vi "FieldMain.vi"() -> ()   [LabVIEW 2014]
uses:
  <vilib>/picture/3D Picture Control/Object/Create Object (drawable).vi
  <vilib>/picture/3D Picture Control/Object/Add Object (no reference).vi
  <vilib>/picture/3D Picture Control/NI_3D Picture Control.lvlib
panel:
  in  "Stopp":bool
  out "3D-Bild":refnum<vi>(3d-picture)
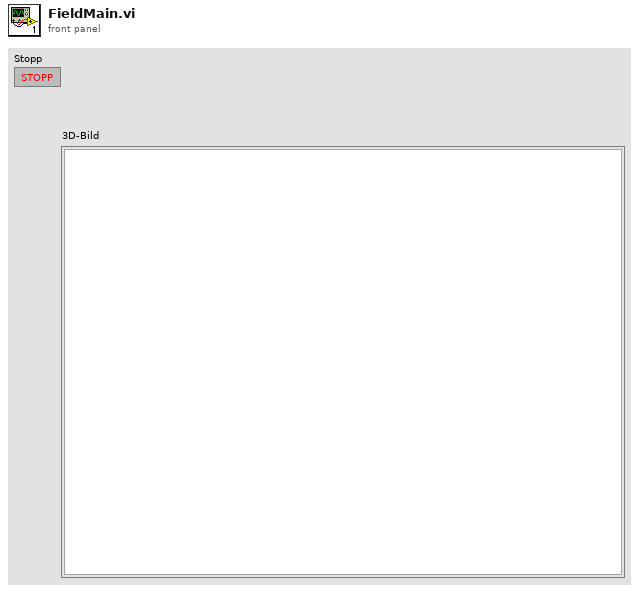
[diagram p1: front panel]
types:
  T1 = cluster{"Red":sgl, "Green":sgl, "Blue":sgl, "Alpha":sgl}
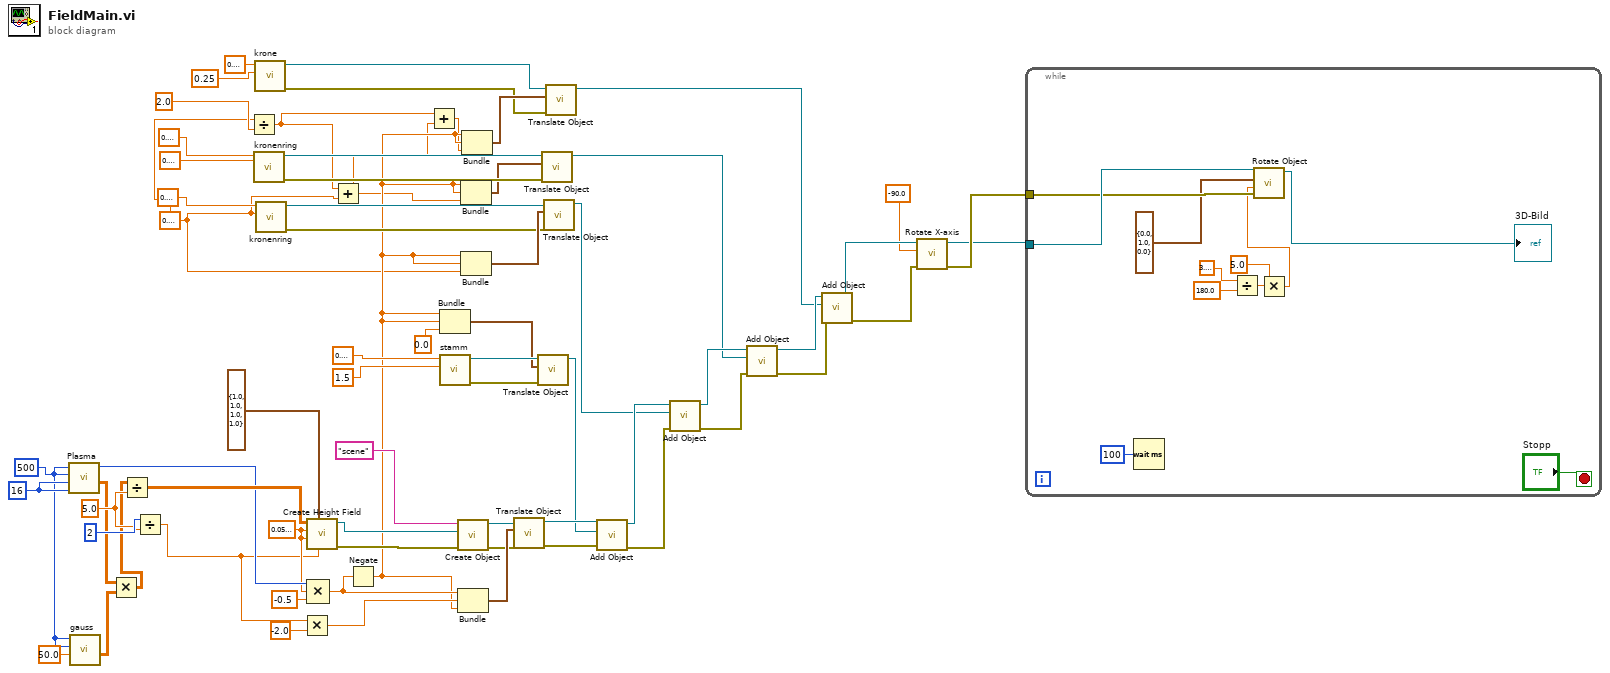
[diagram p0: block diagram]
diagram:
  w12 = sgl 0.6 ("Radius")
  w61 = 16 ("x")
  w59 = sgl 5.0 ("Base Height")
  w57 = sgl 0.05 ("Row Interval")
  w37 = 500
  n1 = call "Plasma.vi"("Periods2"=w61, "Periods1"=w61, "N2"=w37, "N1"=w37) -> ("Array"=w34:dbl[][], "N1 out"=w58:i32)  [unwired: 5 in, 1 out]
  n2 = call "gauss.vi"("w"=50.0, "N2"=w37, "N1"=w37) -> ("Array"=w35:dbl[][])  [unwired: 6 in, 2 out]
  n3 = Multiply(x=w34, y=w35) -> (x*y=w33:dbl[][])
  n4 = Divide(x=w33, y=w59) -> (x/y=w63:dbl[][])
  n5 = Divide(x=2, y=w59) -> (x/y=w27:sgl)
  n6 = Divide(x=w12, y=sgl 2.0) -> (x/y=w1:sgl)
  n7 = call "kronenring.vi"("Height"=sgl 0.6 ("Radius"), "Radius"=sgl 0.3 ("Height")) -> ("error out"=w23:errorcluster, "Scene Object Out"=w22:refnum<vi>)  [unwired: 8 in]
  n8 = call "krone.vi"("Radius"=sgl 0.25, "Height"=sgl 0.7) -> ("Fehler (Ausgang)"=w8:errorcluster, "SceneObject (Ausgang)"=w10:refnum<vi>)  [unwired: 8 in]
  n9 = call "kronenring.vi"("Height"=w12, "Radius"=sgl 0.6 ("Height")) -> ("error out"=w29:errorcluster, "Scene Object Out"=w31:refnum<vi>)  [unwired: 8 in]
  n10 = Multiply(x=w27, y=sgl -2.0) -> (x*y=w51:sgl)
  n11 = call <vilib>:"Create Height Field.vi"("Base Height"=w27, "Color"=T1 {"Red"=1.0, "Green"=1.0, "Blue"=1.0, "Alpha"=1.0}, "Column Interval"=w57, "Row Interval"=w57, "Data"=w63) -> ("error out"=w65:errorcluster, "New Height Field Refnum"=w64:refnum<vi>)  [unwired: 5 in]
  n12 = Compound Arithmetic op=MULTIPLY(w58, w57, sgl -0.5 ("Wert")) -> (w50:sgl)
  n13 = Add(x=w1, y=w12) -> (x+y=w11:sgl)
  n14 = Negate(x=w50) -> (-x=w13:sgl)
  n15 = Add(x=w1, y=w11) -> (x+y=w9:sgl)
  n16 = Bundle(w13, w13, "angle"=0.0) -> (w40:cluster{sgl, sgl, "angle":dbl})  [unwired: 1 in]
  n17 = call "stamm.vi"("Height"=sgl 1.5, "Radius"=sgl 0.2) -> ("Fehler (Ausgang)"=w43:errorcluster, "SceneObject (Ausgang)"=w44:refnum<vi>)  [unwired: 8 in]
  n18 = call-poly <vilib>:"Create Object.vi"("error in (no error)"=w65, "Geometry"=w64, "Name"="scene") -> ("error out"=w45:errorcluster, "Scene:New Object"=w46:refnum<vi>)  [unwired: 7 in]
  n19 = Bundle(w50, w51, w13) -> (w54:cluster{sgl, sgl, sgl})  [unwired: 1 in]
  n20 = Bundle(w13, w13, w11) -> (w21:cluster{sgl, sgl, sgl})  [unwired: 1 in]
  n21 = Bundle(w13, w13, "Radius"=w12) -> (w30:cluster{sgl, sgl, "Radius":sgl})  [unwired: 1 in]
  n22 = Bundle(w13, w13, w9) -> (w14:cluster{sgl, sgl, sgl})  [unwired: 1 in]
  n23 = call <vilib>:"Translate Object.vi"("error in (no error)"=w45, "Translation"=w54, "Scene.Object In"=w46) -> ("error out"=w48:errorcluster, "Scene.Object Out"=w47:refnum<vi>)  [unwired: 7 in]
  n24 = call <vilib>:"Translate Object.vi"("error in (no error)"=w43, "Translation"=w40, "Scene.Object In"=w44) -> ("Scene.Object Out"=w42:refnum<vi>)  [unwired: 7 in, 1 out]
  n25 = call <vilib>:"Translate Object.vi"("error in (no error)"=w23, "Translation"=w21, "Scene.Object In"=w22) -> ("Scene.Object Out"=w17:refnum<vi>)  [unwired: 7 in, 1 out]
  n26 = call <vilib>:"Translate Object.vi"("error in (no error)"=w29, "Translation"=w30, "Scene.Object In"=w31) -> ("Scene.Object Out"=w18:refnum<vi>)  [unwired: 7 in, 1 out]
  n27 = call <vilib>:"Translate Object.vi"("error in (no error)"=w8, "Translation"=w14, "Scene.Object In"=w10) -> ("Scene.Object Out"=w3:refnum<vi>)  [unwired: 7 in, 1 out]
  n28 = call-poly <vilib>:"Add Object.vi"("error in (no error)"=w48, "New Object In"=w42, "Scene Object In"=w47) -> ("error out"=w38:errorcluster, "Scene Object Out"=w39:refnum<vi>)  [unwired: 7 in]
  n29 = call-poly <vilib>:"Add Object.vi"("error in (no error)"=w38, "New Object In"=w18, "Scene Object In"=w39) -> ("error out"=w20:errorcluster, "Scene Object Out"=w19:refnum<vi>)  [unwired: 7 in]
  n30 = call-poly <vilib>:"Add Object.vi"("error in (no error)"=w20, "New Object In"=w17, "Scene Object In"=w19) -> ("error out"=w2:errorcluster, "Scene Object Out"=w4:refnum<vi>)  [unwired: 7 in]
  n31 = call-poly <vilib>:"Add Object.vi"("error in (no error)"=w2, "New Object In"=w3, "Scene Object In"=w4) -> ("error out"=w7:errorcluster, "Scene Object Out"=w6:refnum<vi>)  [unwired: 7 in]
  n32 = call <vilib>:"Rotate X-axis.vi"("error in (no error)"=w7, "angle"=-90.0, "Scene Object In"=w6) -> ("error out"=w53:errorcluster, "Scene Object Out"=w52:refnum<vi>)  [unwired: 7 in]
  n33 = while {
    tunnel: w53 -> [w73]
    tunnel: w52 -> [w74]
    stop <- "Stopp" stop-if-true
    n34 = Wait (ms)(milliseconds to wait=u32 100 ("Zu wartende ms")) -> ()  [unwired: 1 out]
    n35 = Divide(x=3.141592653589793 ("angle"), y=180.0) -> (x/y=w69:dbl)
    n36 = Multiply(x=w69, y=5.0) -> (x*y=w68:dbl)
    n37 = call <vilib>:"Rotate Object.vi"("error in (no error)"=w73, "Angle"=w68, "Axis"=cluster{"X":sgl, "Y":sgl, "Z":sgl} {"X"=0.0, "Y"=1.0, "Z"=0.0}, "Scene.Object In"=w74) -> ("Scene.Object Out"=→"3D-Bild":refnum<vi>)  [unwired: 6 in, 1 out]
  }
